vi "Event MessengerM Channel Wire  -  Async Modules.vi"() -> ()   [LabVIEW 2020]
doc: "This example shows how to specify the receiving event structure on the same Event MessengerM Channel connecting those."
uses:
  672d3064-7071-417b-b93c-895df1d30760.vi
  023db999-cac3-4b1c-b71c-6266668e4539.vi
  53cbacac-594c-4138-abf4-dbf2c683047f.vi
  b9f869d2-90c5-4296-86ac-c51af813fb60.vi
  f4150c67-e98c-4e93-a863-113ea2982431.vi
  80310944-eb72-43fc-8926-2008ae03a107.vi
panel:
  in  "self":string caption="self subchannel"
  out "Result":dbl
  in  "Max Button":bool
  in  "Multiply Button":bool
  in  "Add Button":bool
  in  "Elements":dbl[](array[numeric])
  in  "Abort Button":bool
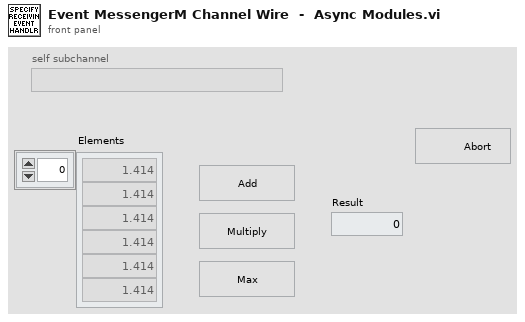
[diagram p1: front panel]
types:
  T1 = cluster{"self":string, "subs":map{string, string}}
  T2 = typedef "Event MessengerM-c(str,var).lvlib/))Channel.ctl" = refnum<queue>
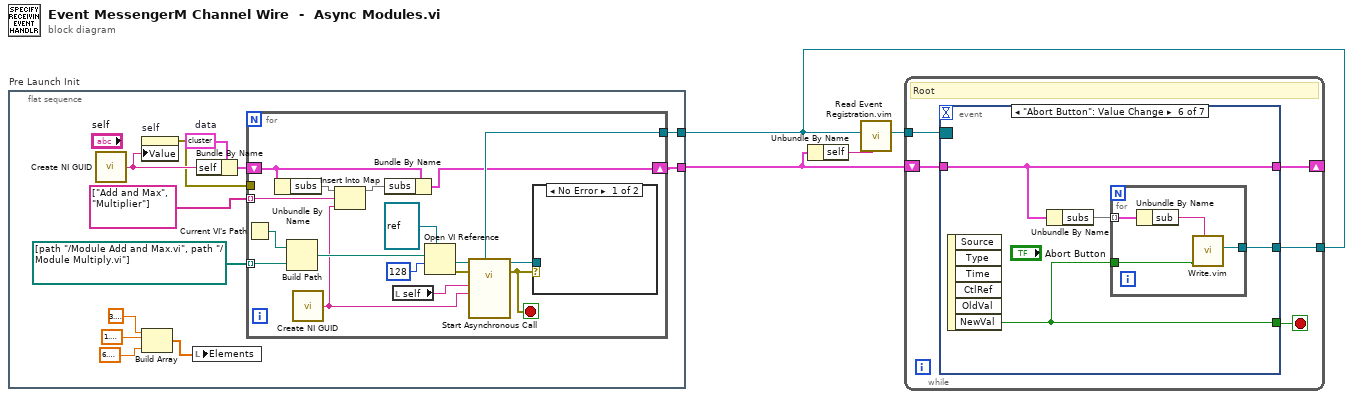
[diagram p0: block diagram]
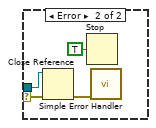
[diagram p2: hidden frame]
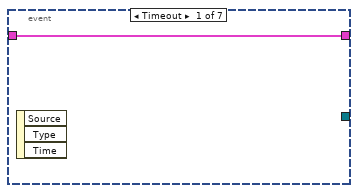
[diagram p3: hidden frame]
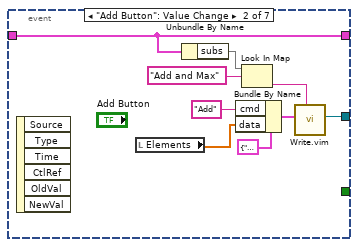
[diagram p4: hidden frame]
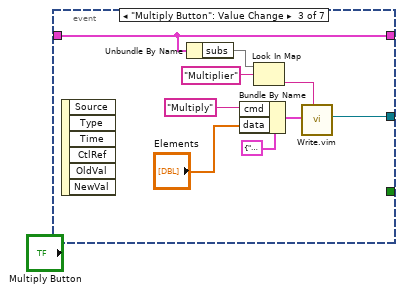
[diagram p5: hidden frame]
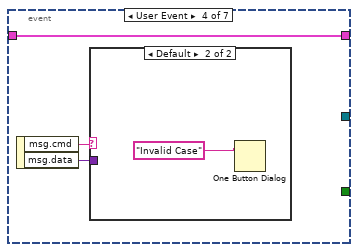
[diagram p6: hidden frame]
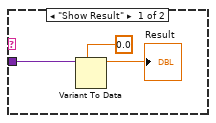
[diagram p7: hidden frame]
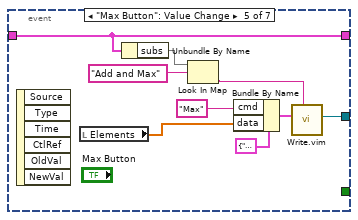
[diagram p8: hidden frame]
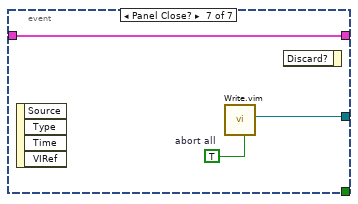
[diagram p9: hidden frame]
diagram:
  n1 = flat-sequence "Pre Launch Init" {
    tunnel: [w12] -> w2
    tunnel: w3 -> [w15]
    frame #0 {
      w14 = T1 {"self"="", "subs"={}}  # data
      n2 = call <vilib>:"Create NI GUID.vi"() -> ("NI GUID"=w6:string)
      n3 = property on="self" class="Str"("Value"=w6) -> (error out=w5:errorcluster)  [unwired: 2 in, 1 out]
      n4 = Build Array(3.141592653589793, 1.5707963267948966, 6.283185307179586) -> (w10:dbl[])
      n5 = local write "Elements"(w10) -> ()
      n6 = Bundle By Name(cluster=w14, "self"=w6) -> (w13:T1)
      n7 = for {
        tunnel: path[] [path "../Module Add and Max.vi", path "../Module Multiply.vi"] -> [w29] mode=indexing
        tunnel: w15 -> [w30]
        tunnel: string[] ["Add and Max", "Multiplier"] -> [w28] mode=indexing
        shift-right: [w20] -> w12
        shift-left: w13 -> [w19]
        tunnel: w5 -> [_]
        stop <- w24 stop-if-true
        n8 = Current VI's Path() -> (path=w17:path)
        n9 = Unbundle By Name(w19) -> ("subs"=w18:map{string, string})
        n10 = Build Path(base path=w17, name or relative path=w29) -> (appended path=w26:path)
        n11 = call <vilib>:"Create NI GUID.vi"() -> ("NI GUID"=w22:string)
        n12 = Insert Into Map(map in=w18, key=w28, value=w22) -> (map out=w21:map{string, string})  [unwired: 2 out]
        n13 = Bundle By Name(cluster=w19, "subs"=w21) -> (w20:T1)
        n14 = local read "self"() -> (w27:string)
        n15 = Open VI Reference(type specifier VI Refnum (for type only)=refnum<vi> refnum, vi path=w26, options=128) -> (vi reference=w31:refnum<vi>, error out=w25:errorcluster)  [unwired: 3 in]
        n16 = call-by-ref "Start Asynchronous Call"(reference=w31, error in=w25, "channel"=w30, "self"=w22, "caller"=w27) -> (reference out=w23:refnum<vi>, error out=w24:errorcluster)  [unwired: 9 in]
        n17 = case shown="No Error" w24 {
          selector: w24 -> [_ w37]
          tunnel: w23 -> [_ w36]
          frame No Error {
          }
          frame Error {
            n18 = Close Reference(reference=w36, error in (no error)=w37) -> (error out=w34:errorcluster)
            n19 = Stop(stop? (T)=TRUE) -> ()
            n20 = call <vilib>:"Simple Error Handler.vi"("error in (no error)"=w34) -> ()  [unwired: 4 in, 5 out]
          }
        }
      }
    }
  }
  n21 = Unbundle By Name(w2) -> ("self"=w1:string)
  n22 = call "Read Event Registration.vim"("subchannel"=w1, "channel"=w3) -> ("event registration refnum"=w4:refnum<event-registration>)  [unwired: 9 in]
  n23 = while {
    tunnel: w4 -> [w41]
    tunnel: [w40] -> w3
    shift-right: [w38] -> _
    shift-left: w2 -> [w39]
    stop <- w42 stop-if-true
    # "Root"
    n24 = event shown="[5] \"Abort Button\": Value Change" {
      selector: w41 -> [_ _ _ _ _ _ _]
      dyn-events: _ -> [_ _ _ _ _ _ _]
      timeout: _ -> [_ _ _ _ _ _ _]
      tunnel: [_ _ _ _ _ w79 _] -> w42
      tunnel: [_ w50 w61 _ w72 w80 w88] -> w40
      tunnel: w39 -> [w43 w45 w54 w62 w69 w81 w87]
      tunnel: [w43 w45 w54 w62 w69 w81 w87] -> w38
      event Timeout {
        n25 = event-data() -> ()  [unwired: 1 in, 3 out]
      }
      event "Add Button": Value Change {
        n26 = event-data() -> ()  [unwired: 1 in, 6 out]
        n27 = local read "Elements"() -> (w46:dbl[])
        n28 = Unbundle By Name(w45) -> ("subs"=w44:map{string, string})
        n29 = Bundle By Name(cluster=cluster{"cmd":string, "data":variant} {"cmd"="", "data"=variant} ("element"), "cmd"="Add", "data"=w46) -> (w48:cluster{"cmd":string, "data":variant})
        n30 = Look In Map(map=w44, key="Add and Max") -> (value=w51:string)  [unwired: 1 in, 1 out]
        n31 = call "Write.vim"("subchannel"=w51, "element"=w48) -> ("channel"=w50:T2)  [unwired: 8 in, 1 out]
      }
      event "Multiply Button": Value Change {
        n32 = event-data() -> ()  [unwired: 1 in, 6 out]
        n33 = Unbundle By Name(w54) -> ("subs"=w53:map{string, string})
        n34 = Bundle By Name(cluster=cluster{"cmd":string, "data":variant} {"cmd"="", "data"=variant} ("element"), "cmd"="Multiply", "data"="Elements") -> (w56:cluster{"cmd":string, "data":variant})
        n35 = Look In Map(map=w53, key="Multiplier") -> (value=w59:string)  [unwired: 1 in, 1 out]
        n36 = call "Write.vim"("subchannel"=w59, "element"=w56) -> ("channel"=w61:T2)  [unwired: 8 in, 1 out]
      }
      event User Event {
        n37 = event-data() -> ("msg.cmd"=w64:string, "msg.data"=w63:variant)  [unwired: 1 in]
        n38 = case shown="Default" w64 {
          tunnel: w63 -> [w67 _]
          frame "Show Result" {
            n39 = Variant To Data(type=0.0, Variant=w67) -> (data=→"Result":dbl)  [unwired: 1 in, 1 out]
          }
          frame Default {
            n40 = One Button Dialog(message="Invalid Case") -> ()  [unwired: 1 in, 1 out]
          }
        }
      }
      event "Max Button": Value Change {
        n41 = event-data() -> ()  [unwired: 1 in, 6 out]
        n42 = local read "Elements"() -> (w71:dbl[])
        n43 = Unbundle By Name(w69) -> ("subs"=w70:map{string, string})
        n44 = Look In Map(map=w70, key="Add and Max") -> (value=w76:string)  [unwired: 1 in, 1 out]
        n45 = Bundle By Name(cluster=cluster{"cmd":string, "data":variant} {"cmd"="", "data"=variant} ("element"), "cmd"="Max", "data"=w71) -> (w74:cluster{"cmd":string, "data":variant})
        n46 = call "Write.vim"("subchannel"=w76, "element"=w74) -> ("channel"=w72:T2)  [unwired: 8 in, 1 out]
      }
      event "Abort Button": Value Change {
        n47 = event-data() -> ("NewVal"=w79:bool)  [unwired: 1 in, 5 out]
        n48 = Unbundle By Name(w81) -> ("subs"=w78:map{string, string})
        n49 = for {
          tunnel: w78 -> [w85] mode=indexing
          tunnel: [w83] -> w80
          tunnel: w79 -> [w82]
          n50 = Unbundle By Name(w85) -> ("sub"=w84:string)
          n51 = call "Write.vim"("subchannel"=w84, "abort sub (F)"=w82) -> ("channel"=w83:T2)  [unwired: 8 in, 1 out]
        }
      }
      event Panel Close? {
        w86 = TRUE  # abort all
        n52 = event-data() -> ()  [unwired: 1 in, 4 out]
        n53 = call "Write.vim"("abort all (F)"=w86) -> ("channel"=w88:T2)  [unwired: 9 in, 1 out]
        n54 = event-data() -> ()  [unwired: 2 in, 1 out]
      }
    }
  }
